vi "GrabToTrackerOnly.vi"(0 "IMAQ Refnum in":refnum<k11>, 2 "Framerate":i32, 3 "QTrk Instance":T5, 4 "ROIs":cluster{"X":i32, "Y":i32}[](array[cluster]), 6 "stop":refnum<vi>, 7 "Type":T4, 9 "#ROI":u32, 10 "Output Queue":refnum<queue>, 12 "ResultManager":T3, 13 "ROI Size":cluster{"X":i32, "Y":i32}) -> ()   [LabVIEW 2011]
uses:
  qtrk/QTrkLVBinding/QTrkInstance.ctl
  Main/Typedefs/CmdEnum_CameraFrameType.ctl
  qtrk/QTrkLVBinding/ResultManagerInstance.ctl
  Main/Typedefs/CmdData_NewFrame.ctl
  <vilib>/vision/Image Controls.llb/IMAQ Image.ctl
  Main/Motors/MotorPosType.ctl
  Main/Typedefs/XYf.ctl
  qtrk/QTrkLVBinding/QTrkLocalizationJob.ctl
  qtrk/QTrkLVBinding/XYZf.ctl
  qtrk/QTrkLVBinding/QTrkPixelDataType.ctl
  qtrk/QTrkLVBinding/QTrkDLL.vi
  Main/GlobalVariables.vi
panel:
  out "Current Position":T1
  out "widths":u32[](array[numeric])
  in  "Stop2":bool
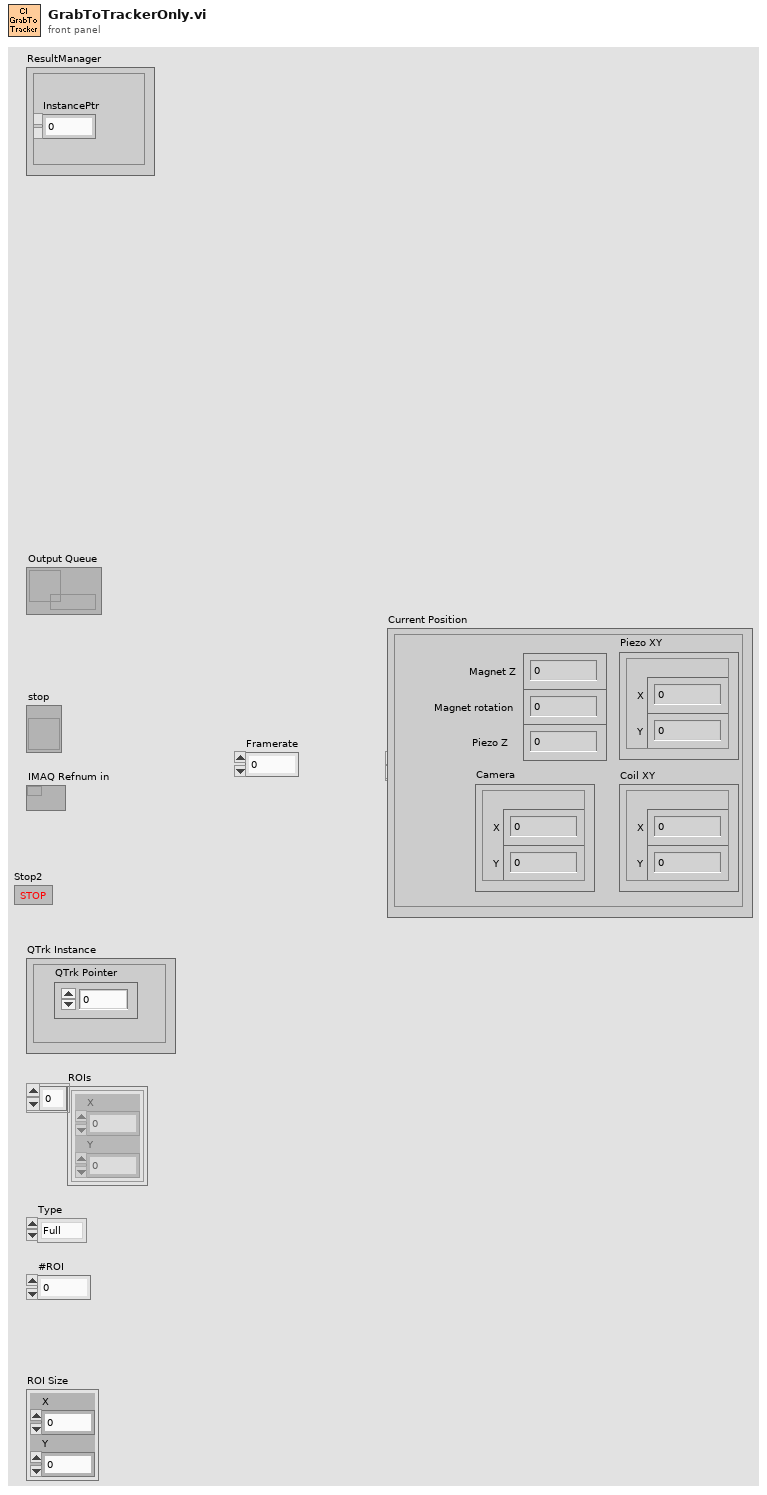
[diagram p1: front panel]
types:
  T1 = typedef "MotorPosType.ctl" = cluster{"Magnet Z":dbl, "Magnet rotation":dbl, "Camera":T2, "Piezo XY":T2, "Piezo Z":dbl, "Coil XY":T2}
  T2 = typedef "XYf.ctl" = cluster{"X":sgl, "Y":sgl}
  T3 = typedef "ResultManagerInstance.ctl" = cluster{"InstancePtr":u64}
  T4 = typedef "CmdEnum_CameraFrameType.ctl" = enum16{"Full", "HardwareROI", "EndGrabMarker"}
  T5 = typedef "QTrkInstance.ctl" = cluster{"QTrk Pointer":u64}
  T6 = typedef "MotorStateType.ctl" = cluster{"Enabled?":bool, "Current Position":T1, "Update counter":i32}
  T7 = typedef "IMAQ Image.ctl" = refnum<image>
  T8 = typedef "QTrkPixelDataType.ctl" = enum16{"QTrkU8", "QTrkU16", "QTrkFloat"}
  T9 = typedef "QTrkComputedSettings.ctl" = cluster{"QTrk Settings":T10, "Derived settings":cluster{"ZLUT Radial Steps":i32, "ZLUT Angular Steps":i32, "ZLUT Max Radius":sgl, "QI Radial Steps":i32, "QI Angular Steps\nPer Quadrant":i32, "QI Max Radius":sgl}}
  T10 = typedef "QTrkSettings.ctl" = cluster{"Image width":i32, "Image height":i32, "Number of threads (CPU based)":i32, "CUDA Device":i32, "COM Background correction factor":sgl, "ZLUT MinRadius":sgl, "ZLUT Radial sample density":sgl, "ZLUT Angular sample density":sgl, "ZLUT ROI Coverage":sgl, "QI Iterations":i32, "QI MinRadius":sgl, "QI Radial sample density":sgl, "QI Angular sample density":sgl, "QI ROI Coverage":sgl, "QI Angular Step \nIteration Factor":sgl, "XCOR Profile Length":i32, "XCOR Profile Width":i32, "XCOR Iterations":i32, "Gaussian 2D Fit Iterations":i32, "Gaussian 2D Sigma (pixels)":sgl, "Downsample":i32}
  T11 = enum32{"Map Pixel Pointer", "Unmap Pixel Pointer", "Get Pixels Infos"}
  T12 = typedef "QTrkLocalizationJob.ctl" = cluster{"Frame#":u32, "Timestamp":u32, "ZLUT Index / bead#":i32, "Initial guess":T13}
  T13 = typedef "XYZf.ctl" = cluster{"X":sgl, "Y":sgl, "Z":sgl}
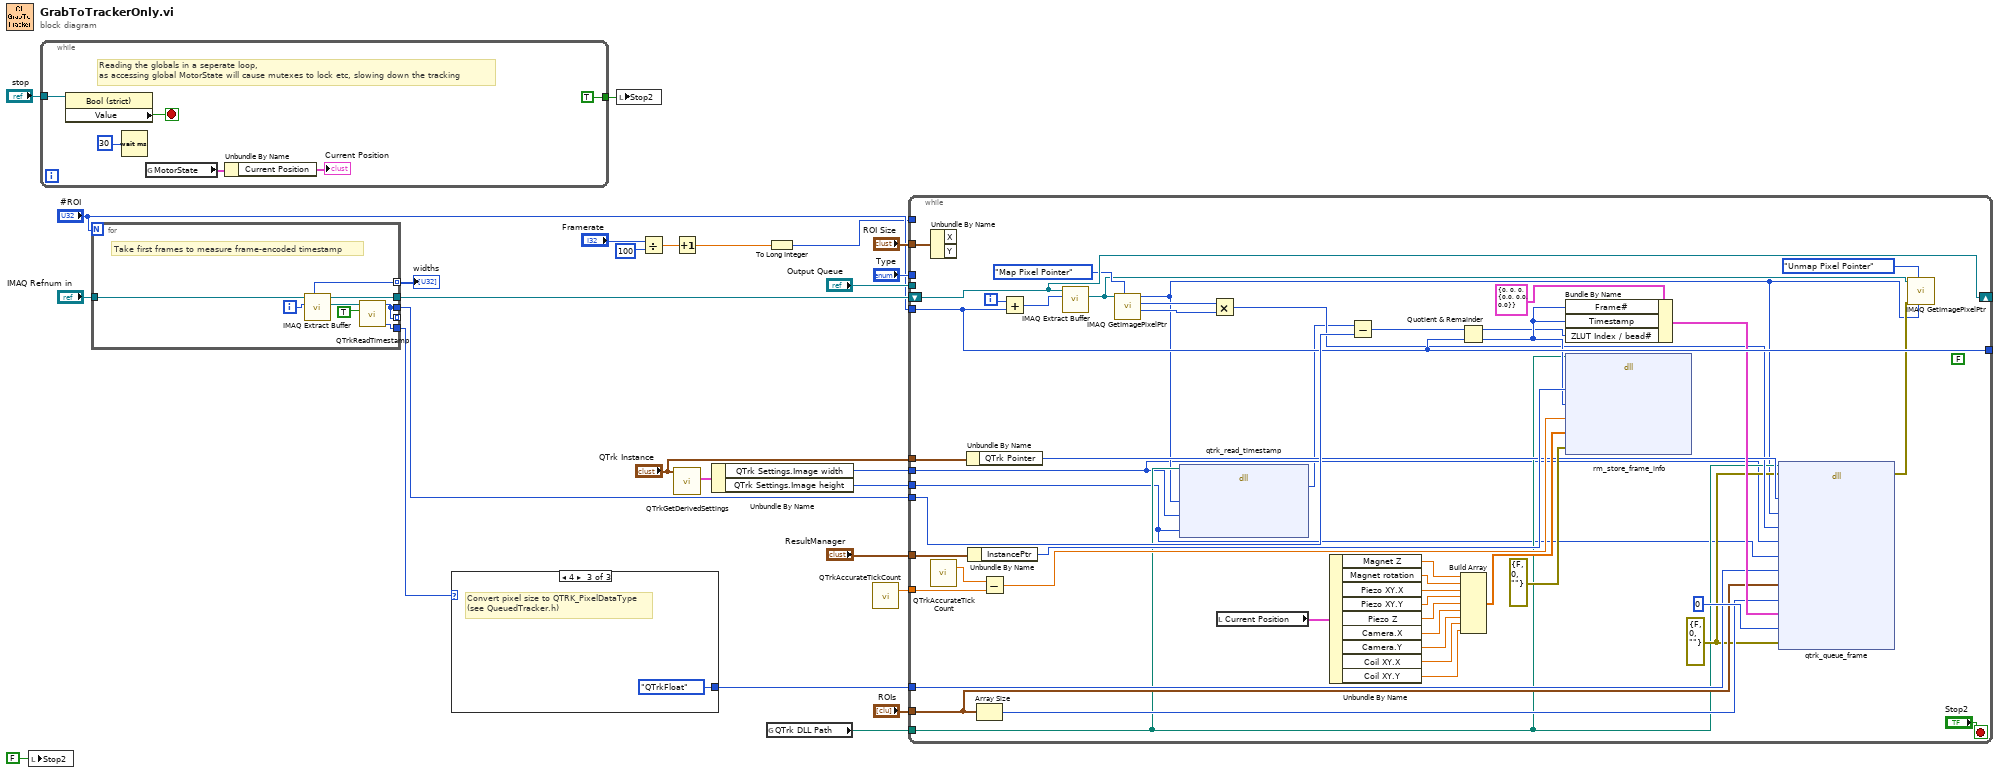
[diagram p0: block diagram]
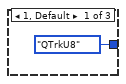
[diagram p2: hidden frame]
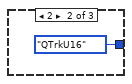
[diagram p3: hidden frame]
diagram:
  n1 = local write "Stop2"(FALSE ("Stop2")) -> ()
  n2 = while {
    tunnel: "stop" -> [w31]
    tunnel: [TRUE ("Stop2")] -> w16
    stop <- w32 stop-if-true
    # "Reading the globals in a seperate loop, \nas accessing global MotorState will cause mutexes to lock etc, slowing down the tracking"
    n3 = property on="Property Node" class="Bool (strict)"(reference=w31) -> ("Value"=w32:bool)  [unwired: 1 in, 2 out]
    n4 = Wait (ms)(milliseconds to wait=u32 30) -> ()  [unwired: 1 out]
    n5 = global read "GlobalVariables.vi" "MotorState"() -> (w28:T6)
    n6 = Unbundle By Name(w28) -> ("Current Position"=→"Current Position":T1)
  }
  n7 = for {
    N: "#ROI" -> [_]
    tunnel: "IMAQ Refnum in" -> [w40]
    tunnel: [w39] -> w19
    tunnel: [w37] -> w8
    tunnel: [w37] -> _ mode=indexing
    tunnel: [w36] -> w9 mode=indexing
    tunnel: [w33] -> w1
    i -> [w38]
    # "Take first frames to measure frame-encoded timestamp"
    n8 = call <vilib>:"IMAQ Extract Buffer.vi"("Buffer to extract"=w38, "IMAQ Session In"=w40) -> ("Image Out"=w34:T7, "IMAQ Session Out"=w39:refnum<k11>, "Actual Width"=w36:u32)  [unwired: 4 in, 3 out]
    n9 = call "QTrkReadTimestamp.vi"("Use QTrk code?"=TRUE, "Image"=w34) -> ("Pixel Size (Bytes)"=w33:i32, "timestamp"=w37:u32)  [unwired: 8 in]
  }
  "widths" <- w9
  n10 = case shown="4" w1 {
    tunnel: [QTrkPixelDataType."QTrkU8" ("Pixel data type") QTrkPixelDataType."QTrkU16" ("Pixel data type") QTrkPixelDataType."QTrkFloat" ("Pixel data type")] -> w2
    frame 1, Default {
    }
    frame 2 {
    }
    frame 4 {
      # "Convert pixel size to QTRK_PixelDataType\n(see QueuedTracker.h)"
    }
  }
  n11 = local write "Stop2"(w16) -> ()
  n12 = Divide(x="Framerate", y=100) -> (x/y=w12:dbl)
  n13 = Increment(x=w12) -> (x+1=w11:dbl)
  n14 = call "QTrkGetDerivedSettings.vi"("QTrk Instance"="QTrk Instance") -> ("Derived settings"=w6:T9)  [unwired: 5 in, 5 out]
  n15 = Unbundle By Name(w6) -> ("QTrk Settings.Image width"=w5:i32, "QTrk Settings.Image height"=w4:i32)
  n16 = global read "QTrkDLL.vi" "QTrk DLL Path"() -> (w3:path)
  n17 = To Long Integer(number=w11) -> (32bit integer=w10:i32)
  n18 = call "QTrkAccurateTickCount.vi"() -> ("tick count (ms)"=w21:dbl)  [unwired: 2 in, 1 out]
  n19 = while {
    tunnel: "Output Queue" -> [_]
    shift-right: [w91] -> _
    shift-left: w19 -> [w91]
    tunnel: "QTrk Instance" -> [w60]
    tunnel: [w83] -> _
    tunnel: w21 -> [w89]
    tunnel: "ROIs" -> [w55]
    tunnel: "ResultManager" -> [w67]
    tunnel: "Type" -> [_]
    tunnel: w8 -> [w88]
    tunnel: "ROI Size" -> [w87]
    tunnel: "#ROI" -> [w83]
    tunnel: w10 -> [_]
    tunnel: w5 -> [w46]
    tunnel: w4 -> [w45]
    tunnel: w3 -> [w48]
    tunnel: w2 -> [w53]
    i -> [w84]
    stop <- "Stop2" stop-if-true
    w52 = errorcluster {"status"=FALSE, "code"=0, "source"=""} ("error in (no error)")
    (unwired) FALSE ("Clear first 4 bytes in frame? (F)")
    n20 = Unbundle By Name(w87) -> ()  [unwired: 2 out]
    n21 = call "QTrkAccurateTickCount.vi"() -> ("tick count (ms)"=w90:dbl)  [unwired: 2 in, 1 out]
    n22 = Unbundle By Name(w60) -> ("QTrk Pointer"=w59:u64)
    n23 = Unbundle By Name(w67) -> ("InstancePtr"=w66:u64)
    n24 = Array Size(array=w55) -> (size(s)=w54:i32)
    n25 = Subtract(x=w90, y=w89) -> (x-y=w65:dbl)
    n26 = Add(x=w84, y=w83) -> (x+y=w82:u32)
    n27 = call <vilib>:"IMAQ Extract Buffer.vi"("Buffer to extract"=w82, "IMAQ Session In"=w91) -> ("Image Out"=w51:T7)  [unwired: 4 in, 5 out]
    n28 = call "IMAQ GetImagePixelPtr"("Function"=T11."Map Pixel Pointer", "Image"=w51) -> ("Pixel Size (Bytes)"=w57:i32, "LineWidth(Pixels)"=w58:i32, "Pixel Pointer out"=w47:u64)  [unwired: 4 in, 3 out]
    n29 = dll-call lib="D:/jcnossen1/cudaqi-tracker/bin/jtrkcuda-labview.dll" fn="qtrk_read_timestamp"(path in=w48, "imageptr"=w47, "width"=w46, "height"=w45) -> ("timestamp"=w44:u32)  [unwired: 5 in, 2 out]
    n30 = Multiply(x=w58, y=w57) -> (x*y=w56:i32)
    n31 = local read "Current Position"() -> (w68:T1)
    n32 = Unbundle By Name(w68) -> ("Magnet Z"=w77:dbl, "Magnet rotation"=w76:dbl, "Piezo XY.X"=w75:sgl, "Piezo XY.Y"=w74:sgl, "Piezo Z"=w73:dbl, "Camera.X"=w72:sgl, "Camera.Y"=w71:sgl, "Coil XY.X"=w70:sgl, "Coil XY.Y"=w69:sgl)
    n33 = Subtract(x=w44, y=w88) -> (x-y=w86:u32)
    n34 = Quotient & Remainder(x=w86, y=w83) -> (x-y*floor(x/y)=w61:u32, floor(x/y)=w62:u32)
    n35 = Build Array(w77, w76, w75, w74, w73, w72, w71, w70, w69) -> (w64:dbl[])
    n36 = Bundle By Name(cluster=T12 {"Frame#"=0, "Timestamp"=0, "ZLUT Index / bead#"=0, "Initial guess"={"X"=0.0, "Y"=0.0, "Z"=0.0}} ("jobInfo"), "Frame#"=w62, "Timestamp"=w62, "ZLUT Index / bead#"=w61) -> (w78:T12)
    n37 = dll-call lib="D:/jcnossen1/cudaqi-tracker/bin/jtrk-labview.dll" fn="rm_store_frame_info"(path in=w48, "resultmanager"=w66, "frame"=w62, "timestamp"=w65, "columns"=w64, "error"=errorcluster {"status"=FALSE, "code"=0, "source"=""}) -> ()  [unwired: 8 in, 2 out]
    n38 = dll-call lib="D:/jcnossen1/cudaqi-tracker/bin/jtrk-labview.dll" fn="qtrk_queue_frame"(path in=w48, error in=w52, "tracker"=w59, "image"=w47, "pitch"=w56, "width"=w46, "height"=w45, "format"=w53, "positions"=w55, "numROI"=w54, "jobInfo"=w78, "flags"=0, "err"=w52) -> (error out=w49:errorcluster)  [unwired: 13 in, 1 out]
    n39 = call "IMAQ GetImagePixelPtr"("Pixel Pointer in"=w47, "Function"=T11."Unmap Pixel Pointer", "error in (no error)"=w49, "Image"=w51) -> ()  [unwired: 2 in, 6 out]
  }
